vi "Autonomous Independent.vi"() -> ()   [LabVIEW 2018]
doc: "This VI is called when autonomous begins, and will automatically be terminated when autonomous ends. You can carry out timed or sensor driven robot movement independently without needing to return to the caller."
uses:
  <vilib>/Analysis/baseanly.llb/Mean (DBL).vi
  <vilib>/Rock Robotics/WPI/Utilities/WPI_GetSetVariantRefNum.vi
  <vilib>/Rock Robotics/Network Tables/NT Read Number.vi
  <vilib>/Rock Robotics/Network Tables/NT Write Numeric Array.vi
  <vilib>/Rock Robotics/Network Tables/NT Write String.vi
  Robot Global Data.vi
  <vilib>/Rock Robotics/WPI/RobotDrive/WPI_RobotDriveArcadeDrive_Standard(NoSaturation).vi
  <vilib>/Rock Robotics/Network Tables/NT Write Number.vi
  <vilib>/Analysis/NI_AALBase.lvlib
panel:
  in  "Array of robot movements":T1(array[cluster])=[{"X Joystick Value"=0.39393939393939403, "Y Joystick Value"=0.0, "Delay (sec)"=1.0, "Movement Name"="turn"}, {"X Joystick Value"=-0.3737373737373737, "Y Joystick Value"=0.0, "Delay (sec)"=1.0, "Movement Name"="turn back"}] {"Y Joystick Value" scale=1.0..-1.0; "X Joystick Value" scale=-1.0..1.0}
  out "Current Movement, for debugging":T2 {"Y Joystick Value" scale=1.0..-1.0; "X Joystick Value" scale=-1.0..1.0}
  # "Be sure to right-click and choose Data Operations>>Make Current Value default if you want to save the array values with the VI"
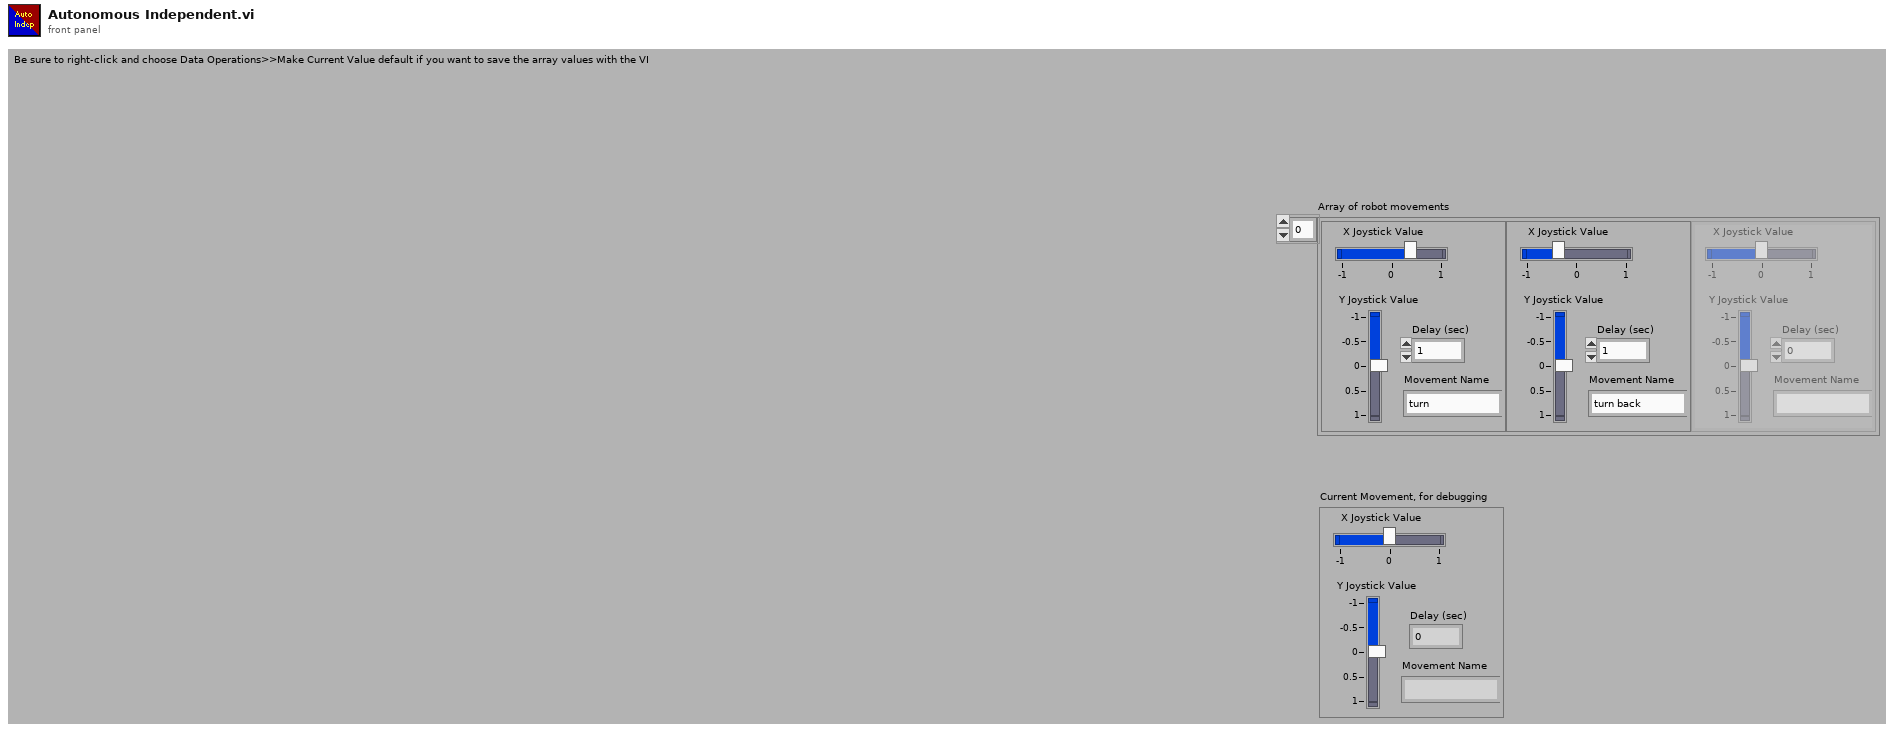
[diagram p1: front panel]
types:
  T1 = cluster{"X Joystick Value":dbl, "Y Joystick Value":dbl, "Delay (sec)":dbl, "Movement Name":string}[]
  T2 = cluster{"X Joystick Value":dbl, "Y Joystick Value":dbl, "Delay (sec)":dbl, "Movement Name":string}
  T3 = typedef "WPI_JoystickDevRef.ctl" = cluster{"Device":T4}
  T4 = typedef "WPI_JoystickDeviceEnum.ctl" = enum16{"USB 0", "USB 1", "USB 2", "USB 3", "USB 4", "USB 5"}
  T5 = typedef "WPI_RobotDriveDevRef.ctl" = cluster{"DevStatus":errorcluster, "Motors[]":T6[], "Square Inputs":bool, "Max Output":dbl}
  T6 = typedef "WPI_MotorControlDeviceRef.ctl" = cluster{"DeviceStatus":errorcluster, "Type":T7, "PWM":cluster{"PWM Channel":T8, "DeadBand":T9}, "CAN":cluster{"Device Number":u8, "SetOutput VI Ref":variant, "GetOutput VI Ref":variant, "Enable VI Ref":variant, "Disable VI Ref":variant, "Data":variant}, "Invert":bool, "DIO PWM":cluster{"PWM \"Enable\" Channel":T8, "DIOChannel":T10, "PWM Rate":dbl}}
  T7 = typedef "WPI_MotorControlType.ctl" = enum16{"PWM", "CAN", "DIO PWM"}
  T8 = typedef "FPGA_DIOPWMChannel.ctl" = enum8{"PWM 0", "PWM 1", "PWM 2", "PWM 3", "PWM 4", "PWM 5", "PWM 6", "PWM 7", "PWM 8", "PWM 9", "PWM MXP 0", "PWM MXP 1", "PWM MXP 2", "PWM MXP 3", "PWM MXP 4", "PWM MXP 5", "PWM MXP 6", "PWM MXP 7", "PWM MXP 8", "PWM MXP 9", "Invalid"}
  T9 = typedef "WPI_PWMDeadband.ctl" = cluster{"Name":string, "maxPositivePwm":i32, "minPositivePwm":i32, "centerPwm":i32, "maxNegativePwm":i32, "minNegativePwm":i32, "angularRange":u16}
  T10 = typedef "FPGA_DIOChannel.ctl" = enum8{"DIO 0", "DIO 1", "DIO 2", "DIO 3", "DIO 4", "DIO 5", "DIO 6", "DIO 7", "DIO 8", "DIO 9", "DIO MXP 0", "DIO MXP 1", "DIO MXP 2", "DIO MXP 3", "DIO MXP 4", "DIO MXP 5", "DIO MXP 6", "DIO MXP 7", "DIO MXP 8", "DIO MXP 9", "DIO MXP 10", "DIO MXP 11", "DIO MXP 12", "DIO MXP 13", "DIO MXP 14", "DIO MXP 15", "SPI Port CS1", "SPI Port CS2", "SPI Port CS3", "SPI Port MISO", "SPI Port MOSI", "Invalid"}
  T11 = typedef "WPI_AnalogChannelDevRef.ctl" = cluster{"DevStatus":errorcluster, "Analog Channel":T12}
  T12 = typedef "FPGA_AIChannel.ctl" = enum8{"AI 0", "AI 1", "AI 2", "AI 3", "AI MXP 0", "AI MXP 1", "AI MXP 2", "AI MXP 3", "Invalid"}
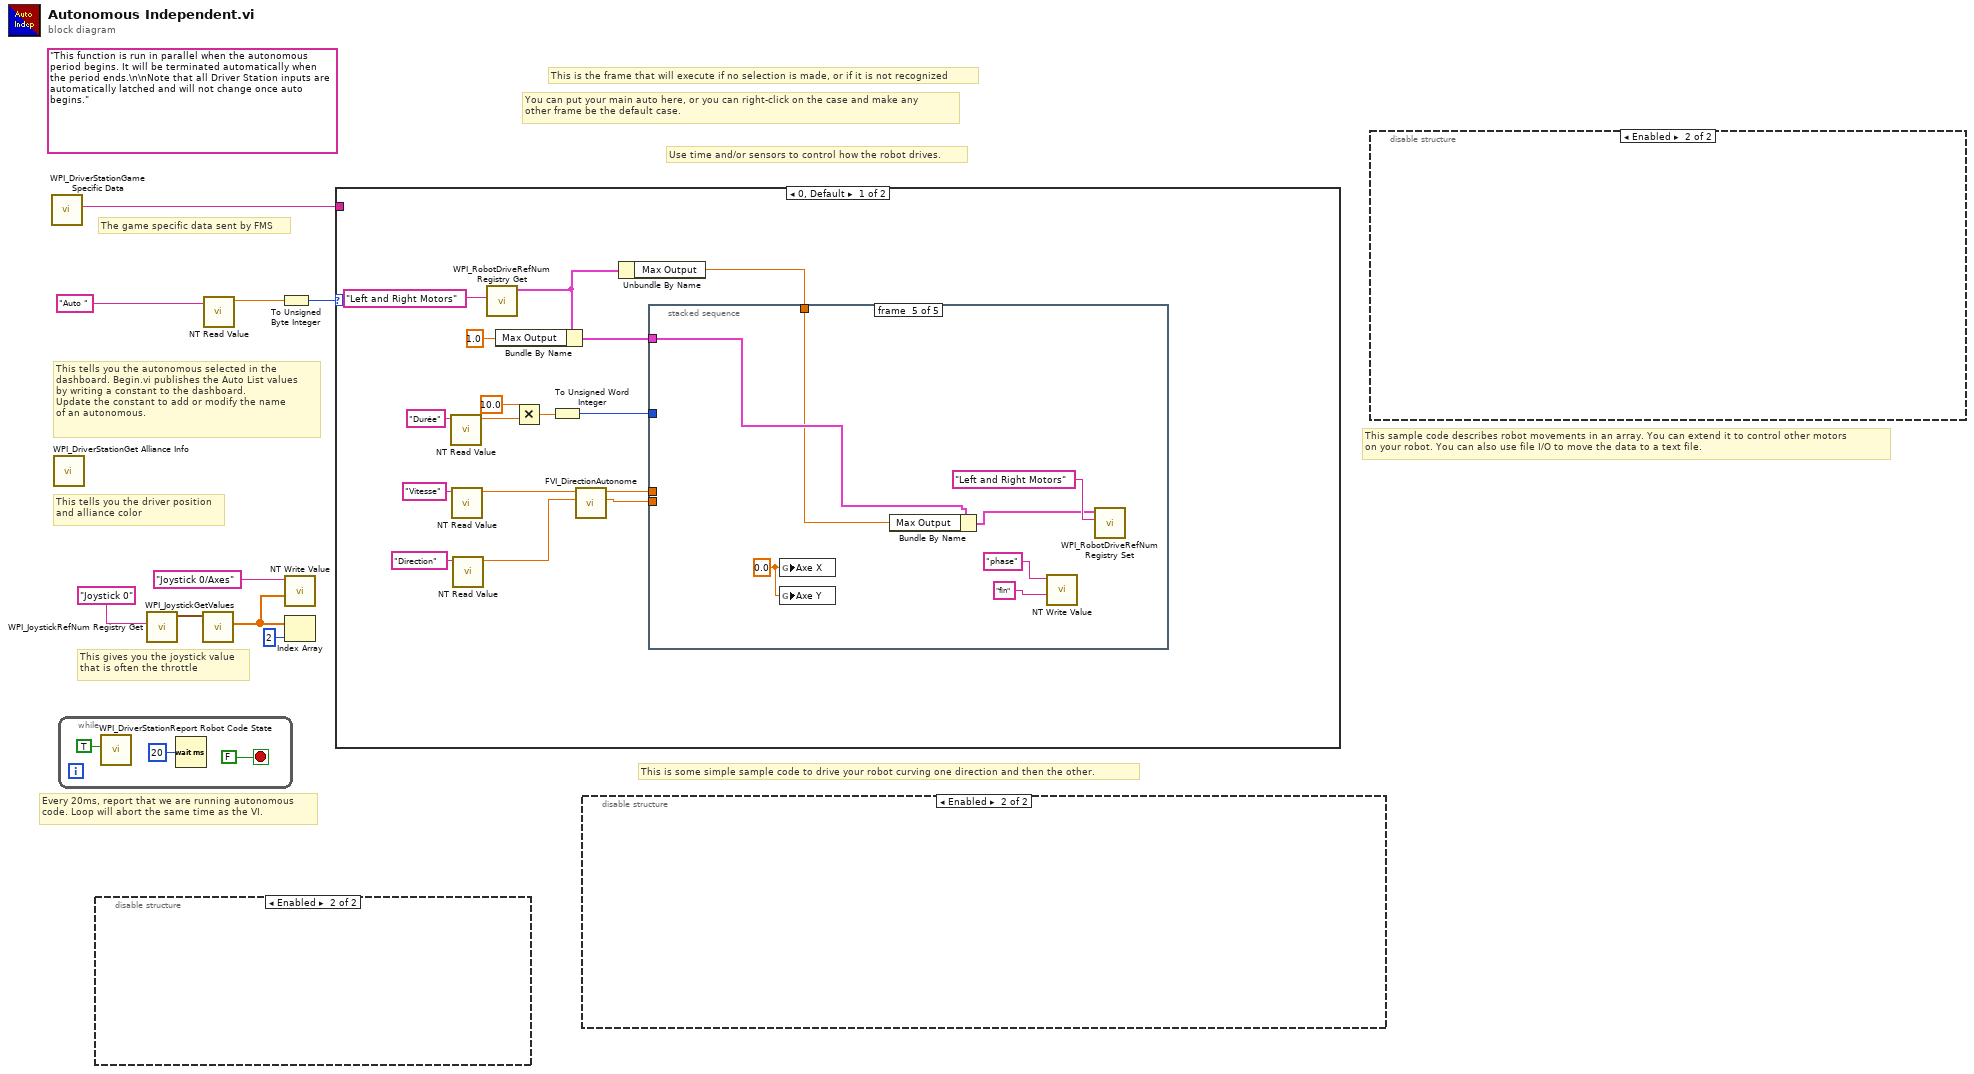
[diagram p0: block diagram]
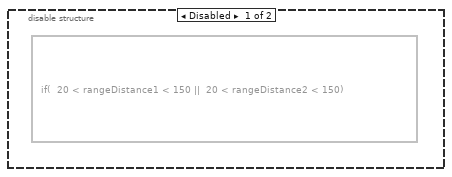
[diagram p2: hidden frame]
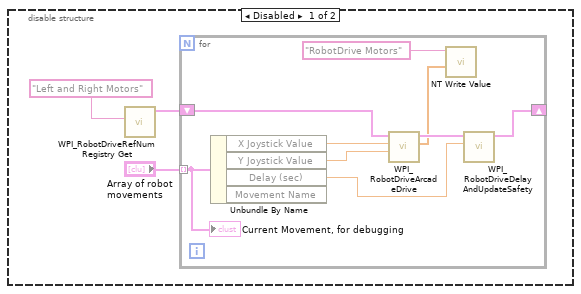
[diagram p3: hidden frame]
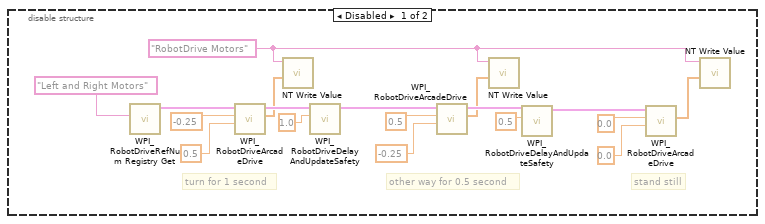
[diagram p4: hidden frame]
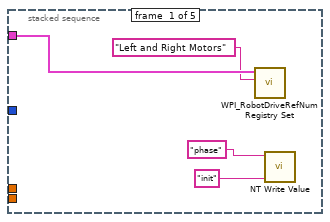
[diagram p5: hidden frame]
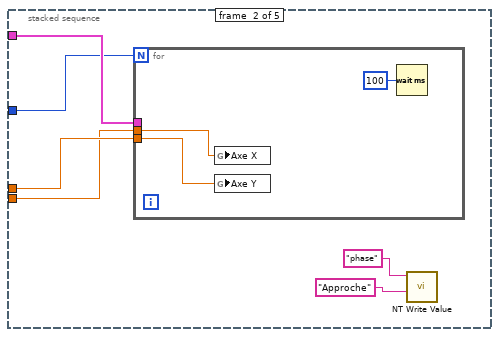
[diagram p6: hidden frame]
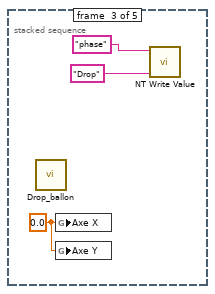
[diagram p7: hidden frame]
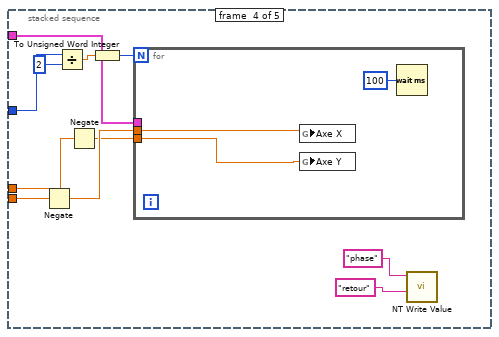
[diagram p8: hidden frame]
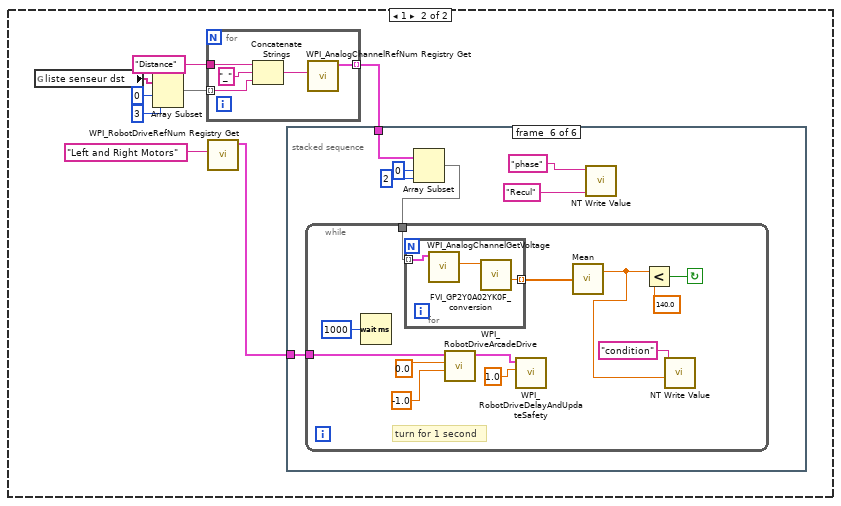
[diagram p9: hidden frame]
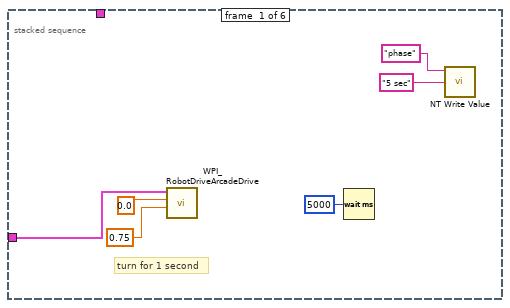
[diagram p10: hidden frame]
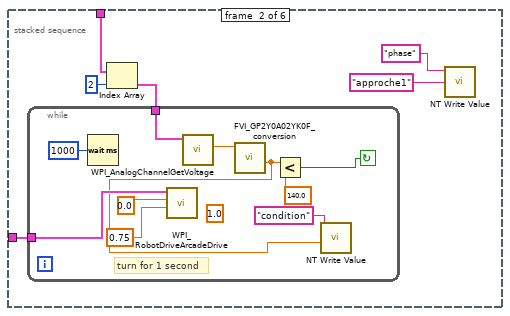
[diagram p11: hidden frame]
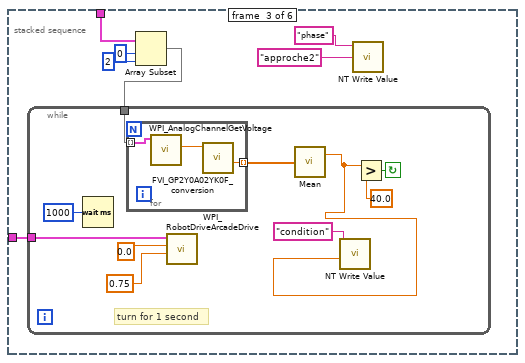
[diagram p12: hidden frame]
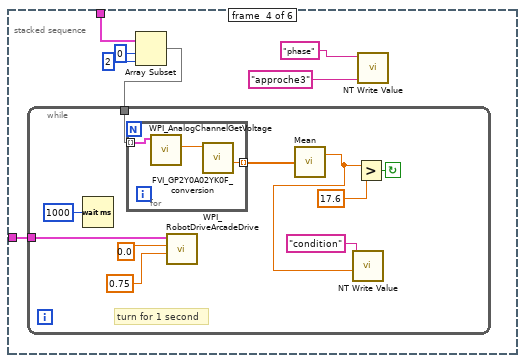
[diagram p13: hidden frame]
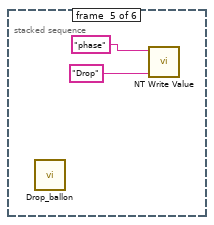
[diagram p14: hidden frame]
diagram:
  (unwired) "This function is run in parallel when the autonomous period begins. It will be terminated automatically when the period ends.\n\nNote that all Driver Station inputs are automatically latched and will not change once auto begins."
  # "You can put your main auto here, or you can right-click on the case and make any\nother frame be the default case."
  # "This is the frame that will execute if no selection is made, or if it is not recognized"
  # "This is some simple sample code to drive your robot curving one direction and then the other."
  # "This sample code describes robot movements in an array. You can extend it to control other motors\non your robot. You can also use file I/O to move the data to a text file."
  # "The game specific data sent by FMS"
  # "This tells you the autonomous selected in the \ndashboard. Begin.vi publishes the Auto List values\nby writing a constant to the dashboard.\nUpdate the constant to add or modify the name\nof an autonomous."
  # "Every 20ms, report that we are running autonomous\ncode. Loop will abort the same time as the VI."
  # "This gives you the joystick value\nthat is often the throttle"
  # "Use time and/or sensors to control how the robot drives."
  # "This tells you the driver position\nand alliance color"
  n1 = call <vilib>:"WPI_DriverStationGame Specific Data.vi"() -> ("Game Specific Data"=w2:string)  [unwired: 11 in]
  n2 = call <vilib>:"WPI_DriverStationGet Alliance Info.vi"() -> ()  [unwired: 12 out]
  n3 = while {
    stop <- FALSE stop-if-true
    n4 = call <vilib>:"WPI_DriverStationReport Robot Code State.vi"("Autonomous"=TRUE) -> ()  [unwired: 10 in, 1 out]
    n5 = Wait (ms)(milliseconds to wait=u32 20) -> ()  [unwired: 1 out]
  }
  n6 = disable-structure shown="Enabled" {
    frame Disabled {
      n7 = formula code="if(  20 < rangeDistance1 < 150 ||  20 < rangeDistance2 < 150)"() -> ()
    }
    frame Enabled {
    }
  }
  n8 = call <vilib>:"WPI_JoystickRefNum Registry Get.vi"("refnum name"="Joystick 0") -> ("JoystickDevRef"=w8:T3)  [unwired: 1 in, 9 out]
  n9 = call <vilib>:"WPI_JoystickGetValues.vi"("JoystickDevRef"=w8) -> ("Axes"=w4:dbl[])  [unwired: 6 in, 4 out]
  n10 = call-poly <vilib>:"NT Read Value.vi"("Name"="Auto ") -> ("Numeric"=w5:dbl)  [unwired: 9 in, 1 out]
  n11 = To Unsigned Byte Integer(number=w5) -> (unsigned 8bit integer=w1:u8)
  n12 = call-poly <vilib>:"NT Write Value.vi"("Numeric Array"=w4, "Name"="Joystick 0/Axes") -> ()  [unwired: 9 in, 1 out]
  n13 = Index Array(array=w4, index=2) -> ()  [unwired: 1 out]
  n14 = case shown="0, Default" w1 {
    tunnel: w2 -> [_ _]
    frame 0, Default {
      n15 = call-poly <vilib>:"NT Read Value.vi"("Name"="Durée") -> ("Numeric"=w24:dbl)  [unwired: 9 in, 1 out]
      n16 = call-poly <vilib>:"NT Read Value.vi"("Name"="Vitesse") -> ("Numeric"=w20:dbl)  [unwired: 9 in, 1 out]
      n17 = call-poly <vilib>:"NT Read Value.vi"("Name"="Direction") -> ("Numeric"=w19:dbl)  [unwired: 9 in, 1 out]
      n18 = call <vilib>:"WPI_RobotDriveRefNum Registry Get.vi"("refnum name"="Left and Right Motors") -> ("RobotDriveDevRef"=w15:T5)  [unwired: 1 in, 9 out]
      n19 = Bundle By Name(cluster=w15, "Max Output"=1.0) -> (w14:T5)
      n20 = Multiply(x=10.0, y=w24) -> (x*y=w22:dbl)
      n21 = To Unsigned Word Integer(number=w22) -> (unsigned 16bit integer=w21:u16)
      n22 = call "FVI_DirectionAutonome.vi"("Direction"=w19, "vitesse"=w20) -> ("x"=w17:dbl, "y"=w18:dbl)  [unwired: 8 in]
      n23 = Unbundle By Name(w15) -> ("Max Output"=w13:dbl)
      n24 = stacked-sequence {
        tunnel: w14 -> [w32 w38 _ w55 w62]
        tunnel: w21 -> [_ w37 _ w48 _]
        tunnel: w18 -> [_ w36 _ w54 _]
        tunnel: w17 -> [_ w35 _ w53 _]
        tunnel: w13 -> [_ _ _ _ w59]
        frame #0 {
          n25 = call <vilib>:"WPI_RobotDriveRefNum Registry Set.vi"("refnum name"="Left and Right Motors", "RobotDriveDevRef"=w32) -> ()  [unwired: 8 in, 2 out]
          n26 = call-poly <vilib>:"NT Write Value.vi"("String"="init", "Name"="phase") -> ()  [unwired: 9 in, 1 out]
        }
        frame #1 {
          n27 = for {
            N: w37 -> [_]
            tunnel: w38 -> [_]
            tunnel: w36 -> [w39]
            tunnel: w35 -> [w40]
            n28 = global write "Robot Global Data.vi" "Axe X"(w40) -> ()
            n29 = global write "Robot Global Data.vi" "Axe Y"(w39) -> ()
            n30 = Wait (ms)(milliseconds to wait=u32 100) -> ()  [unwired: 1 out]
          }
          n31 = call-poly <vilib>:"NT Write Value.vi"("String"="Approche", "Name"="phase") -> ()  [unwired: 9 in, 1 out]
        }
        frame #2 {
          w42 = 0.0 ("Axe X")
          n32 = call "Drop_ballon.vi"() -> ()  [unwired: 12 in]
          n33 = global write "Robot Global Data.vi" "Axe X"(w42) -> ()
          n34 = global write "Robot Global Data.vi" "Axe Y"(w42) -> ()
          n35 = call-poly <vilib>:"NT Write Value.vi"("String"="Drop", "Name"="phase") -> ()  [unwired: 9 in, 1 out]
        }
        frame #3 {
          n36 = Negate(x=w53) -> (-x=w50:dbl)
          n37 = Divide(x=w48, y=u16 2) -> (x/y=w46:dbl)
          n38 = Negate(x=w54) -> (-x=w49:dbl)
          n39 = To Unsigned Word Integer(number=w46) -> (unsigned 16bit integer=w45:u16)
          n40 = for {
            N: w45 -> [_]
            tunnel: w55 -> [_]
            tunnel: w49 -> [w56]
            tunnel: w50 -> [w57]
            n41 = global write "Robot Global Data.vi" "Axe X"(w57) -> ()
            n42 = global write "Robot Global Data.vi" "Axe Y"(w56) -> ()
            n43 = Wait (ms)(milliseconds to wait=u32 100) -> ()  [unwired: 1 out]
          }
          n44 = call-poly <vilib>:"NT Write Value.vi"("String"="retour", "Name"="phase") -> ()  [unwired: 9 in, 1 out]
        }
        frame #4 {
          w60 = 0.0 ("Axe X")
          n45 = global write "Robot Global Data.vi" "Axe X"(w60) -> ()
          n46 = global write "Robot Global Data.vi" "Axe Y"(w60) -> ()
          n47 = Bundle By Name(cluster=w62, "Max Output"=w59) -> (w61:T5)
          n48 = call-poly <vilib>:"NT Write Value.vi"("String"="fin", "Name"="phase") -> ()  [unwired: 9 in, 1 out]
          n49 = call <vilib>:"WPI_RobotDriveRefNum Registry Set.vi"("refnum name"="Left and Right Motors", "RobotDriveDevRef"=w61) -> ()  [unwired: 8 in, 2 out]
        }
      }
    }
    frame 1 {
      n50 = global read "Robot Global Data.vi" "liste senseur dst"() -> (w70:string[])
      n51 = Array Subset(array=w70, index=0, length=3) -> (w71:string[])
      n52 = for {
        tunnel: "Distance" -> [w164]
        tunnel: w71 -> [w162] mode=indexing
        tunnel: [w160] -> w66 mode=indexing
        n53 = Concatenate Strings(w164, "_" ("string"), w162) -> (w161:string)
        n54 = call <vilib>:"WPI_AnalogChannelRefNum Registry Get.vi"("refnum name"=w161) -> ("AIDeviceRef"=w160:T11)  [unwired: 9 in, 1 out]
      }
      n55 = call <vilib>:"WPI_RobotDriveRefNum Registry Get.vi"("refnum name"="Left and Right Motors") -> ("RobotDriveDevRef"=w72:T5)  [unwired: 1 in, 9 out]
      n56 = stacked-sequence {
        tunnel: w72 -> [w79 w85 w102 w122 _ w144]
        tunnel: w66 -> [_ w84 w101 w121 _ w143]
        frame #0 {
          # "turn for 1 second"
          n57 = call-poly <vilib>:"WPI_RobotDriveArcadeDrive.vi"("Y axis value"=0.75 ("X axis value"), "X axis value"=0.0, "RobotDriveDevRef"=w79) -> ()  [unwired: 1 in, 8 out]
          n58 = Wait (ms)(milliseconds to wait=u32 5000) -> ()  [unwired: 1 out]
          n59 = call-poly <vilib>:"NT Write Value.vi"("String"="5 sec", "Name"="phase") -> ()  [unwired: 9 in, 1 out]
        }
        frame #1 {
          n60 = Index Array(array=w84, index=2) -> (element=w82:T11)
          n61 = while {
            tunnel: w85 -> [w92]
            tunnel: w82 -> [w90]
            stop <- w88 continue-if-true
            (unwired) 1.0 ("Delay (s)")
            # "turn for 1 second"
            n62 = Wait (ms)(milliseconds to wait=u32 1000) -> ()  [unwired: 1 out]
            n63 = call-poly <vilib>:"WPI_RobotDriveArcadeDrive.vi"("Y axis value"=0.75 ("X axis value"), "X axis value"=0.0, "RobotDriveDevRef"=w92) -> ()  [unwired: 1 in, 8 out]
            n64 = call <vilib>:"WPI_AnalogChannelGetVoltage.vi"("AIDeviceRef"=w90) -> ("Voltage"=w91:dbl)  [unwired: 8 in, 2 out]
            n65 = call "FVI_GP2Y0A02YK0F_conversion.vi"("Voltage"=w91) -> ("x-y"=w86:dbl)  [unwired: 10 in]
            n66 = Less?(x=w86, y=140.0) -> (x < y?=w88:bool)
            n67 = call-poly <vilib>:"NT Write Value.vi"("Numeric"=w86, "Name"="condition") -> ()  [unwired: 9 in, 1 out]
          }
          n68 = call-poly <vilib>:"NT Write Value.vi"("String"="approche1", "Name"="phase") -> ()  [unwired: 9 in, 1 out]
        }
        frame #2 {
          n69 = Array Subset(array=w101, index=0, length=2) -> (w98:T11[])
          n70 = while {
            tunnel: w102 -> [w109]
            tunnel: w98 -> [w106]
            stop <- w107 continue-if-true
            # "turn for 1 second"
            n71 = Wait (ms)(milliseconds to wait=u32 1000) -> ()  [unwired: 1 out]
            n72 = for {
              tunnel: w106 -> [w114] mode=indexing
              tunnel: [w113] -> w105 mode=indexing
              n73 = call <vilib>:"WPI_AnalogChannelGetVoltage.vi"("AIDeviceRef"=w114) -> ("Voltage"=w115:dbl)  [unwired: 8 in, 2 out]
              n74 = call "FVI_GP2Y0A02YK0F_conversion.vi"("Voltage"=w115) -> ("x-y"=w113:dbl)  [unwired: 10 in]
            }
            n75 = call-poly <vilib>:"WPI_RobotDriveArcadeDrive.vi"("Y axis value"=0.75 ("X axis value"), "X axis value"=0.0, "RobotDriveDevRef"=w109) -> ()  [unwired: 1 in, 8 out]
            n76 = call-poly <vilib>:"Mean.vi"("X"=w105) -> ("mean"=w103:dbl)  [unwired: 1 out]
            n77 = call-poly <vilib>:"NT Write Value.vi"("Numeric"=w103, "Name"="condition") -> ()  [unwired: 9 in, 1 out]
            n78 = Greater?(x=w103, y=40.0) -> (0:w107:bool)
          }
          n79 = call-poly <vilib>:"NT Write Value.vi"("String"="approche2", "Name"="phase") -> ()  [unwired: 9 in, 1 out]
        }
        frame #3 {
          n80 = Array Subset(array=w121, index=0, length=2) -> (w118:T11[])
          n81 = while {
            tunnel: w122 -> [w129]
            tunnel: w118 -> [w126]
            stop <- w127 continue-if-true
            # "turn for 1 second"
            n82 = Wait (ms)(milliseconds to wait=u32 1000) -> ()  [unwired: 1 out]
            n83 = for {
              tunnel: w126 -> [w134] mode=indexing
              tunnel: [w133] -> w125 mode=indexing
              n84 = call <vilib>:"WPI_AnalogChannelGetVoltage.vi"("AIDeviceRef"=w134) -> ("Voltage"=w135:dbl)  [unwired: 8 in, 2 out]
              n85 = call "FVI_GP2Y0A02YK0F_conversion.vi"("Voltage"=w135) -> ("x-y"=w133:dbl)  [unwired: 10 in]
            }
            n86 = call-poly <vilib>:"WPI_RobotDriveArcadeDrive.vi"("Y axis value"=0.75 ("X axis value"), "X axis value"=0.0, "RobotDriveDevRef"=w129) -> ()  [unwired: 1 in, 8 out]
            n87 = call-poly <vilib>:"Mean.vi"("X"=w125) -> ("mean"=w123:dbl)  [unwired: 1 out]
            n88 = call-poly <vilib>:"NT Write Value.vi"("Numeric"=w123, "Name"="condition") -> ()  [unwired: 9 in, 1 out]
            n89 = Greater?(x=w123, y=17.6) -> (0:w127:bool)
          }
          n90 = call-poly <vilib>:"NT Write Value.vi"("String"="approche3", "Name"="phase") -> ()  [unwired: 9 in, 1 out]
        }
        frame #4 {
          n91 = call "Drop_ballon.vi"() -> ()  [unwired: 12 in]
          n92 = call-poly <vilib>:"NT Write Value.vi"("String"="Drop", "Name"="phase") -> ()  [unwired: 9 in, 1 out]
        }
        frame #5 {
          n93 = Array Subset(array=w143, index=0, length=2) -> (w140:T11[])
          n94 = while {
            tunnel: w144 -> [w151]
            tunnel: w140 -> [w150]
            stop <- w147 continue-if-true
            # "turn for 1 second"
            n95 = Wait (ms)(milliseconds to wait=u32 1000) -> ()  [unwired: 1 out]
            n96 = for {
              tunnel: w150 -> [w158] mode=indexing
              tunnel: [w157] -> w149 mode=indexing
              n97 = call <vilib>:"WPI_AnalogChannelGetVoltage.vi"("AIDeviceRef"=w158) -> ("Voltage"=w159:dbl)  [unwired: 8 in, 2 out]
              n98 = call "FVI_GP2Y0A02YK0F_conversion.vi"("Voltage"=w159) -> ("x-y"=w157:dbl)  [unwired: 10 in]
            }
            n99 = call-poly <vilib>:"WPI_RobotDriveArcadeDrive.vi"("Y axis value"=-1.0 ("X axis value"), "X axis value"=0.0, "RobotDriveDevRef"=w151) -> ("RobotDriveDevRef"=w153:T5)  [unwired: 1 in, 7 out]
            n100 = call <vilib>:"WPI_RobotDriveDelayAndUpdateSafety.vi"("Delay (s)"=1.0, "RobotDriveDevRef"=w153) -> ()  [unwired: 8 in, 2 out]
            n101 = call-poly <vilib>:"Mean.vi"("X"=w149) -> ("mean"=w145:dbl)  [unwired: 1 out]
            n102 = Less?(x=w145, y=140.0) -> (x < y?=w147:bool)
            n103 = call-poly <vilib>:"NT Write Value.vi"("Numeric"=w145, "Name"="condition") -> ()  [unwired: 9 in, 1 out]
          }
          n104 = call-poly <vilib>:"NT Write Value.vi"("String"="Recul", "Name"="phase") -> ()  [unwired: 9 in, 1 out]
        }
      }
    }
  }
  n105 = disable-structure shown="Enabled" {
    frame Disabled {
      w166 = "RobotDrive Motors" ("Name")
      # "stand still"
      # "other way for 0.5 second"
      # "turn for 1 second"
      n106 = call <vilib>:"WPI_RobotDriveRefNum Registry Get.vi"("refnum name"="Left and Right Motors") -> ("RobotDriveDevRef"=w182:T5)  [unwired: 1 in, 9 out]
      n107 = call-poly <vilib>:"WPI_RobotDriveArcadeDrive.vi"("Y axis value"=0.5 ("X axis value"), "X axis value"=-0.25, "RobotDriveDevRef"=w182) -> ("Motor Values"=w165:dbl[], "RobotDriveDevRef"=w175:T5)  [unwired: 1 in, 6 out]
      n108 = call-poly <vilib>:"NT Write Value.vi"("Numeric Array"=w165, "Name"=w166) -> ()  [unwired: 9 in, 1 out]
      n109 = call <vilib>:"WPI_RobotDriveDelayAndUpdateSafety.vi"("Delay (s)"=1.0, "RobotDriveDevRef"=w175) -> ("RobotDriveDevRef 2"=w176:T5)  [unwired: 8 in, 1 out]
      n110 = call-poly <vilib>:"WPI_RobotDriveArcadeDrive.vi"("Y axis value"=-0.25 ("X axis value"), "X axis value"=0.5, "RobotDriveDevRef"=w176) -> ("Motor Values"=w167:dbl[], "RobotDriveDevRef"=w177:T5)  [unwired: 1 in, 6 out]
      n111 = call-poly <vilib>:"NT Write Value.vi"("Numeric Array"=w167, "Name"=w166) -> ()  [unwired: 9 in, 1 out]
      n112 = call <vilib>:"WPI_RobotDriveDelayAndUpdateSafety.vi"("Delay (s)"=0.5, "RobotDriveDevRef"=w177) -> ("RobotDriveDevRef 2"=w178:T5)  [unwired: 8 in, 1 out]
      n113 = call-poly <vilib>:"WPI_RobotDriveArcadeDrive.vi"("Y axis value"=0.0 ("X axis value"), "X axis value"=0.0, "RobotDriveDevRef"=w178) -> ("Motor Values"=w168:dbl[])  [unwired: 1 in, 7 out]
      n114 = call-poly <vilib>:"NT Write Value.vi"("Numeric Array"=w168, "Name"=w166) -> ()  [unwired: 9 in, 1 out]
    }
    frame Enabled {
    }
  }
  n115 = disable-structure shown="Enabled" {
    frame Disabled {
      n116 = call <vilib>:"WPI_RobotDriveRefNum Registry Get.vi"("refnum name"="Left and Right Motors") -> ("RobotDriveDevRef"=w184:T5)  [unwired: 1 in, 9 out]
      n117 = for {
        shift-right: [w192] -> _
        shift-left: w184 -> [w193]
        tunnel: "Array of robot movements" -> [w188] mode=indexing
        n118 = Unbundle By Name(w188) -> ("X Joystick Value"=w191:dbl, "Y Joystick Value"=w190:dbl, "Delay (sec)"=w189:dbl)  [unwired: 1 out]
        n119 = call-poly <vilib>:"WPI_RobotDriveArcadeDrive.vi"("Y axis value"=w190, "X axis value"=w191, "RobotDriveDevRef"=w193) -> ("Motor Values"=w186:dbl[], "RobotDriveDevRef"=w194:T5)  [unwired: 1 in, 6 out]
        n120 = call-poly <vilib>:"NT Write Value.vi"("Numeric Array"=w186, "Name"="RobotDrive Motors") -> ()  [unwired: 9 in, 1 out]
        n121 = call <vilib>:"WPI_RobotDriveDelayAndUpdateSafety.vi"("Delay (s)"=w189, "RobotDriveDevRef"=w194) -> ("RobotDriveDevRef 2"=w192:T5)  [unwired: 8 in, 1 out]
        "Current Movement, for debugging" <- w188
      }
    }
    frame Enabled {
    }
  }
